vi "UpdateMatlabBoundControl.vi"(9 "name":string, 10 "Control":refnum<vi>, 11 "ExpID":string) -> ()   [LabVIEW 2017]
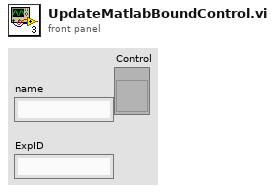
[diagram p1: front panel]
types:
  T1 = typedef "ControlValueChangeEventBindingType.ctl" = cluster{"Control":refnum<vi>, "Event Register":refnum<event-registration>, "AllowVariantValues":bool, "Direction":T2, "Requires Update":bool, "Name":string}
  T2 = typedef "MatlabBindingDirectionEnum.ctl" = enum16{"BiDirectional", "FromMatlab", "ToMatlab"}
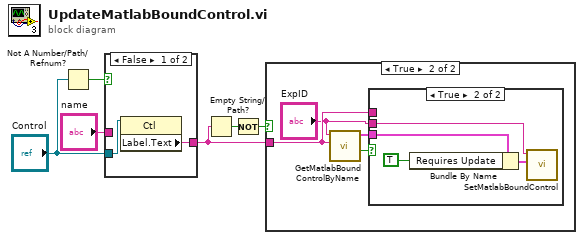
[diagram p0: block diagram]
diagram:
  n1 = Not A Number/Path/Refnum?(number/path/refnum="Control") -> (NaN/Path/Refnum?=w4:bool)
  n2 = case shown="False" w4 {
    tunnel: "name" -> [_ w9]
    tunnel: [w7 w9] -> w2
    tunnel: "Control" -> [w8 _]
    frame False {
      n3 = property class="Ctl"(reference=w8) -> ("Label.Text"=w7:string)  [unwired: 1 in, 2 out]
    }
    frame True {
    }
  }
  n4 = Empty String/Path?(string/path=w2) -> (empty?=w3:bool)
  n5 = Not(x=w3) -> (.not. x?=w1:bool)
  n6 = case shown="True" w1 {
    tunnel: w2 -> [_ w11]
    frame False {
    }
    frame True {
      n7 = call "GetMatlabBoundControlByName.vi"("name"=w11, "ExperimentID"="ExpID") -> ("found"=w13:bool, "Control Binding"=w12:T1)  [unwired: 7 in, 1 out]
      n8 = case shown="True" w13 {
        tunnel: w12 -> [_ w17]
        tunnel: w11 -> [_ _]
        tunnel: "ExpID" -> [_ w15]
        frame False {
        }
        frame True {
          n9 = Bundle By Name(cluster=w17, "Requires Update"=TRUE) -> (w14:T1)
          n10 = call "SetMatlabBoundControl.vi"("Control Binding"=w14, "ExperimentID"=w15) -> ()  [unwired: 10 in]
        }
      }
    }
  }
